vi "UPortal Wait on Load.vi"(8 "error in":errorcluster, 9 "timeout in ms (-1)":i32=5000, 10 "ignore previous (F)":bool=TRUE, 11 "notifier":refnum<notifier>) -> (0 "error out":errorcluster, 1 "time lapsed":u32 format="%.0fms", 2 "notification":string, 3 "notifier out":refnum<notifier>)   [LabVIEW 2020]
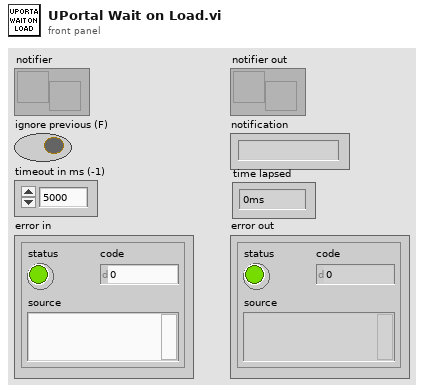
[diagram p1: front panel]
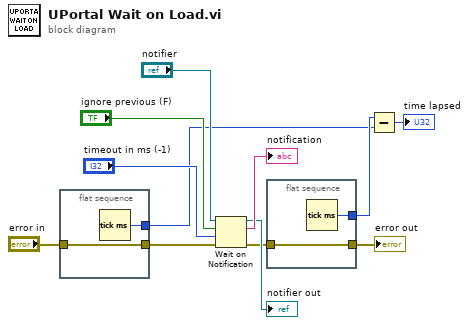
[diagram p0: block diagram]
diagram:
  n1 = flat-sequence {
    tunnel: [w14] -> w2
    tunnel: "error in" -> [w13]
    tunnel: [w13] -> w5
    frame #0 {
      n2 = Tick Count (ms)() -> (millisecond timer value=w14:u32)
    }
  }
  n3 = Wait on Notification(notifier="notifier", ignore previous (F)="ignore previous (F)", timeout in ms (-1)="timeout in ms (-1)", error in (no error)=w5) -> (notifier out=→"notifier out":refnum<notifier>, notification=→"notification":string, error out=w6:errorcluster)  [unwired: 1 out]
  n4 = flat-sequence {
    tunnel: [w16] -> w3
    tunnel: w6 -> [w15]
    tunnel: [w15] -> w4
    frame #0 {
      n5 = Tick Count (ms)() -> (millisecond timer value=w16:u32)
    }
  }
  n6 = Subtract(x=w3, y=w2) -> (x-y=→"time lapsed":u32)
  "error out" <- w4
